vi "4_1.vi"() -> ()   [LabVIEW 2020]
panel:
  in  "Consumer ms":u32
  out "Schieberegler":u8(slide) scale=0.0..100.0
  in  "Producer ms":u32
  out "2":dbl(graph)
  out "Signalverlaufsdiagramm":dbl(graph)
  in  "Stop":bool
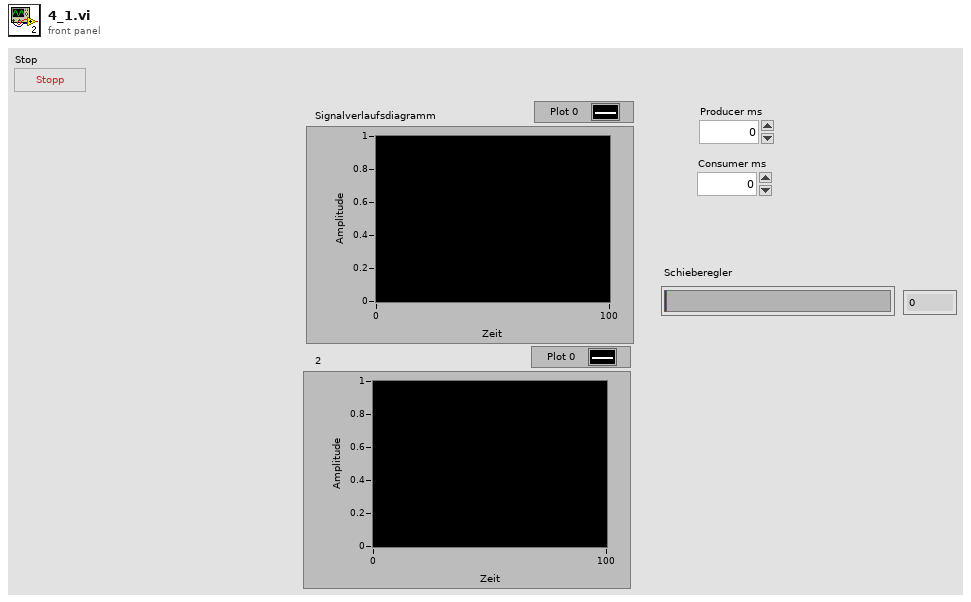
[diagram p1: front panel]
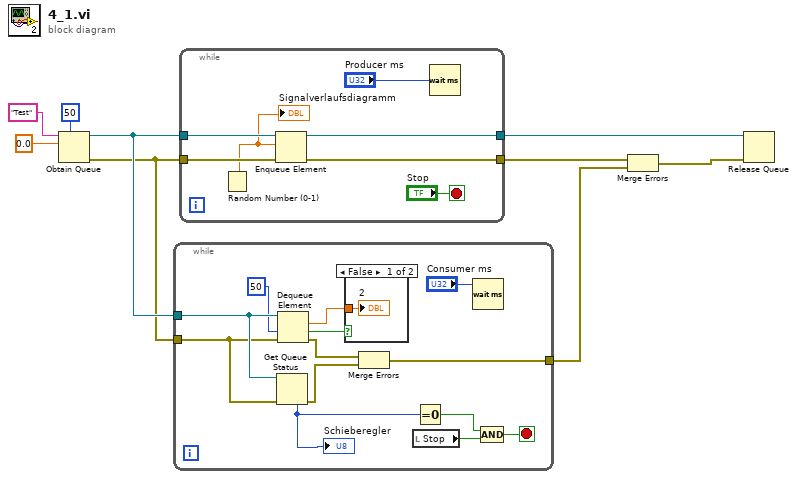
[diagram p0: block diagram]
diagram:
  n1 = Obtain Queue(max queue size (-1, unlimited)=50 ("Maximale Queue-Größe (-1, unbegrenzt)"), name (unnamed)="Test" ("Name (unbenannt)"), element data type=0.0 ("Wert (0 bis 1)")) -> (queue out=w6:refnum<queue>, error out=w5:errorcluster)  [unwired: 2 in, 1 out]
  n2 = while {
    tunnel: w6 -> [w22]
    tunnel: w5 -> [w21]
    tunnel: [w18] -> w3
    stop <- w15 stop-if-true
    n3 = Get Queue Status(queue=w22, error in (no error)=w21) -> (error out=w20:errorcluster, # elements in queue=w11:i32)  [unwired: 1 in, 6 out]
    "Schieberegler" <- w11
    n4 = Dequeue Element(queue=w22, timeout in ms (-1)=50 ("Timeout in ms (-1)"), error in (no error)=w21) -> (element=w13:dbl, timed out?=w12:bool, error out=w19:errorcluster)  [unwired: 1 out]
    n5 = case shown="False" w12 {
      tunnel: w13 -> [w23 _]
      frame False {
        "2" <- w23
      }
      frame True {
      }
    }
    n6 = Merge Errors(w19, w20) -> (w18:errorcluster)
    n7 = local read "Stop"() -> (w17:bool)
    n8 = Equal To 0?(x=w11) -> (x = 0?=w16:bool)
    n9 = Wait (ms)(milliseconds to wait="Consumer ms") -> ()  [unwired: 1 out]
    n10 = Compound Arithmetic op=AND ("Mehrfacharithmetik")(w16, w17) -> (w15:bool)
  }
  n11 = while {
    tunnel: w6 -> [w26]
    tunnel: w5 -> [w30]
    tunnel: [w29] -> w1
    tunnel: [w28] -> w4
    stop <- "Stop" stop-if-true
    n12 = Random Number (0-1)() -> (number: 0 to 1=w25:dbl)
    "Signalverlaufsdiagramm" <- w25
    n13 = Enqueue Element(queue=w26, element=w25, error in (no error)=w30) -> (queue out=w29:refnum<queue>, error out=w28:errorcluster)  [unwired: 1 in, 1 out]
    n14 = Wait (ms)(milliseconds to wait="Producer ms") -> ()  [unwired: 1 out]
  }
  n15 = Merge Errors(w4, w3) -> (w2:errorcluster)
  n16 = Release Queue(queue=w1, error in (no error)=w2) -> ()  [unwired: 1 in, 3 out]
